vi "试验判定.vi"(7 "Result":refnum<vi>, 10 "判定参数":T1, 11 "XY曲线":cluster{"X":dbl[], "Y":dbl[]}[](array[cluster])) -> (2 "判定项长度":i32, 3 "OK？":bool)   [LabVIEW 2020]
uses:
  Global_Variable/A131258.vi
  <userlib>/_MGI/1D Array/MGI Average/MGI Average (DBL[]).vi
panel:
  out "逆向平均值":dbl
  out "正向平均值":dbl
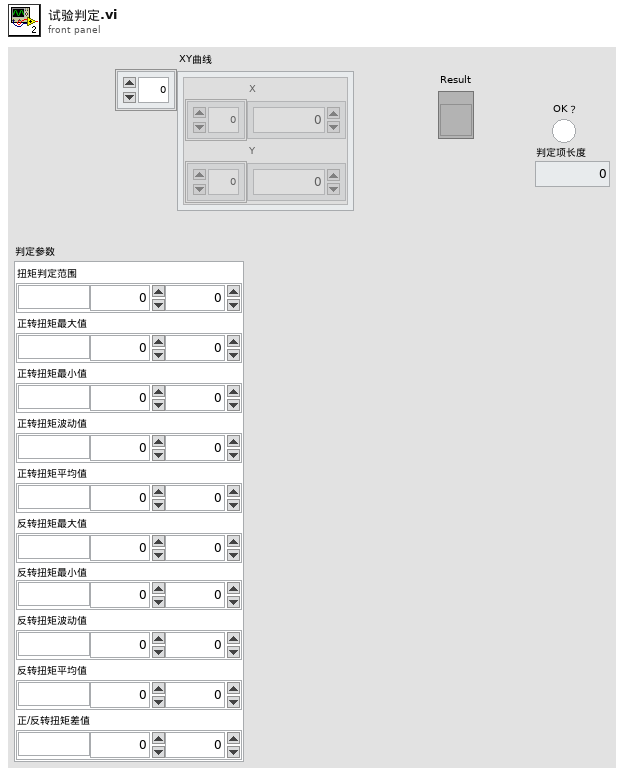
[diagram p1: front panel]
types:
  T1 = cluster{"扭矩判定范围":cluster{"单位":string, "下限":dbl, "上限":dbl}, "正转扭矩最大值":cluster{"单位":string, "下限":dbl, "上限":dbl}, "正转扭矩最小值":cluster{"单位":string, "下限":dbl, "上限":dbl}, "正转扭矩波动值":cluster{"单位":string, "下限":dbl, "上限":dbl}, "正转扭矩平均值":cluster{"单位":string, "下限":dbl, "上限":dbl}, "反转扭矩最大值":cluster{"单位":string, "下限":dbl, "上限":dbl}, "反转扭矩最小值":cluster{"单位":string, "下限":dbl, "上限":dbl}, "反转扭矩波动值":cluster{"单位":string, "下限":dbl, "上限":dbl}, "反转扭矩平均值":cluster{"单位":string, "下限":dbl, "上限":dbl}, "正/反转扭矩差值":cluster{"单位":string, "下限":dbl, "上限":dbl}}
  T2 = cluster{"左平均扭矩":cluster{"正转":dbl, "反转":dbl}, "左矩波动":cluster{"正转":dbl, "反转":dbl}, "左空载":cluster{"正转":dbl, "反转":dbl}, "右平均扭矩":cluster{"正转":dbl, "反转":dbl}, "右扭矩波动":cluster{"正转":dbl, "反转":dbl}, "右空载":cluster{"正转":dbl, "反转":dbl}, "扭矩对称":cluster{"左":dbl, "右":dbl}, "左零点漂移":cluster{"正":dbl, "反":dbl}, "右零点漂移":cluster{"正":dbl, "反":dbl}}
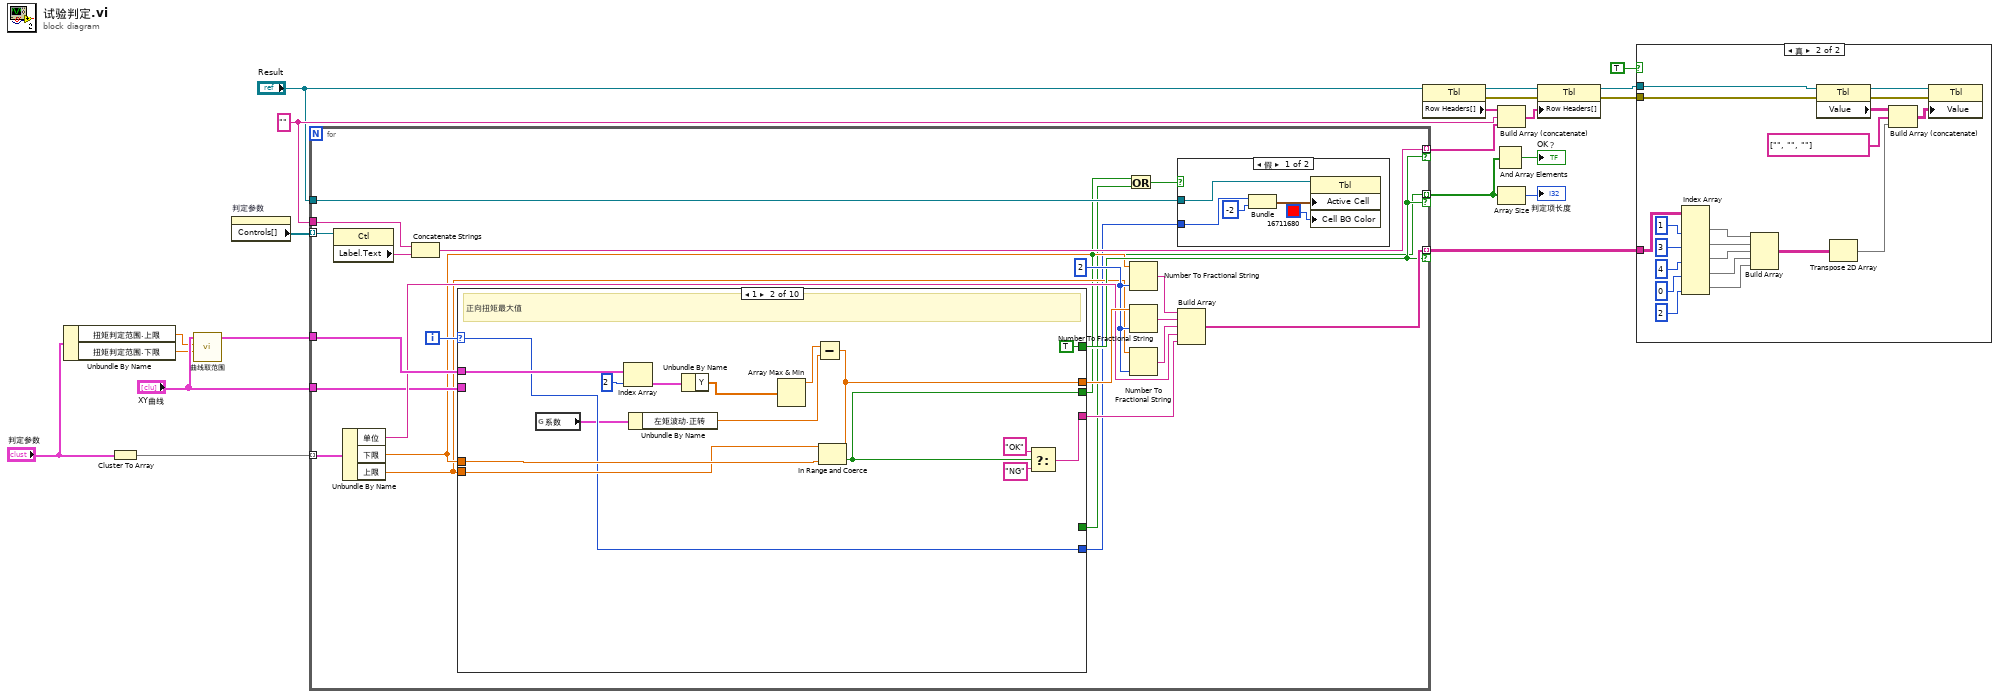
[diagram p0: block diagram]
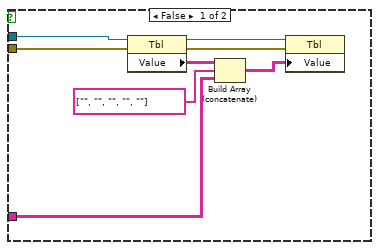
[diagram p2: hidden frame]
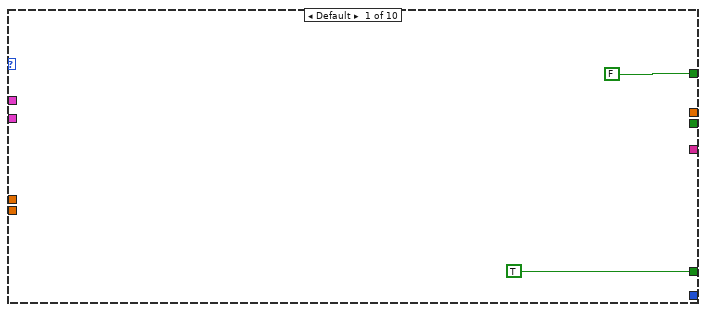
[diagram p4: hidden frame]
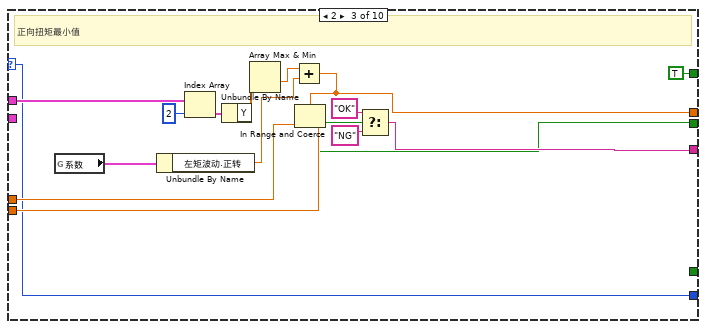
[diagram p5: hidden frame]
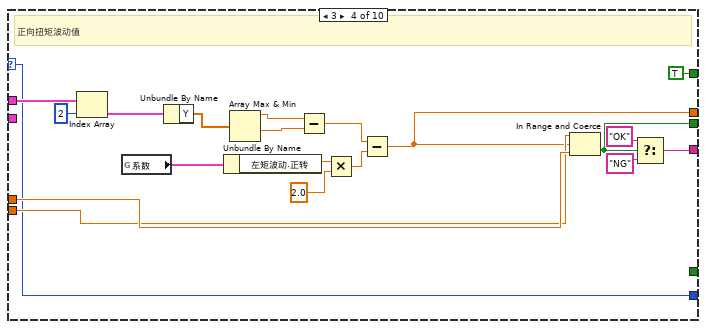
[diagram p6: hidden frame]
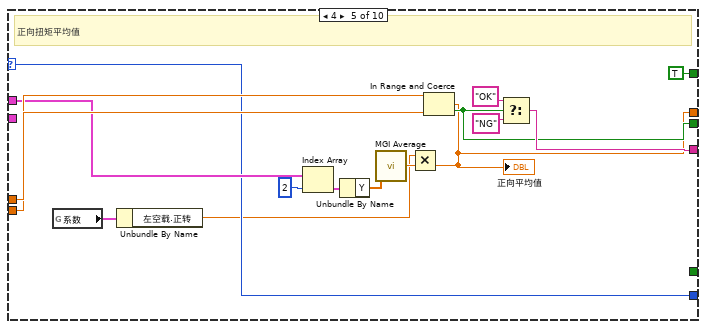
[diagram p7: hidden frame]
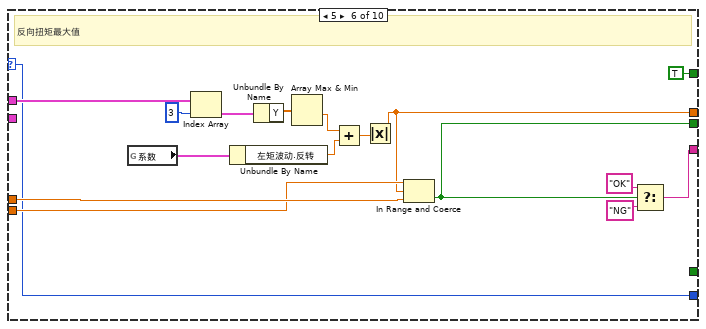
[diagram p8: hidden frame]
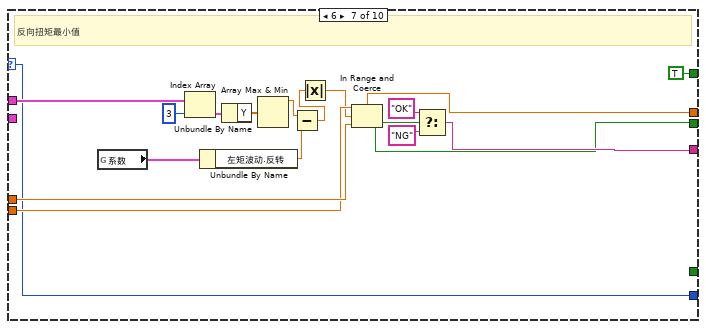
[diagram p9: hidden frame]
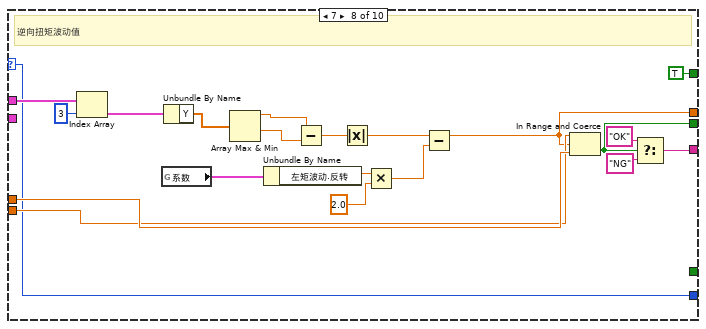
[diagram p10: hidden frame]
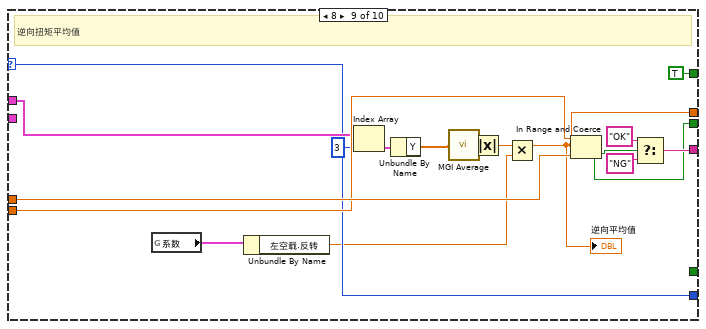
[diagram p11: hidden frame]
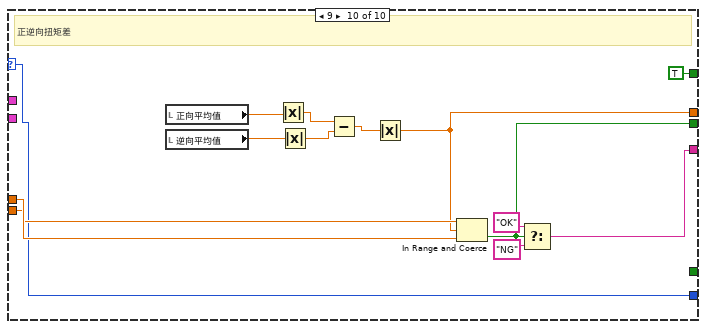
[diagram p12: hidden frame]
diagram:
  w7 = "" ("Label.Text")
  n1 = Unbundle By Name("判定参数") -> ("扭矩判定范围.上限"=w2:dbl, "扭矩判定范围.下限"=w3:dbl)
  n2 = Cluster To Array(cluster="判定参数") -> (array=w21:cluster{"单位":string, "下限":dbl, "上限":dbl}[])
  n3 = call "曲线取范围.vi"("下限"=w3, "上限"=w2, "曲线In"="XY曲线") -> ("曲线Out"=w5:cluster{"X":dbl[], "Y":dbl[]}[])  [unwired: 8 in]
  n4 = property on="判定参数" class="Clust (严格)"() -> ("Controls[]"=w11:refnum<vi>[])  [unwired: 2 in, 2 out]
  n5 = for {
    tunnel: w21 -> [w45] mode=indexing
    tunnel: w11 -> [w43] mode=indexing
    tunnel: w5 -> [w41]
    tunnel: [w25] -> w9 mode=indexing if=w32
    tunnel: [w34] -> w12 mode=indexing if=w32
    tunnel: [w28] -> w14 mode=indexing if=w32
    tunnel: "XY曲线" -> [w31]
    tunnel: w7 -> [w27]
    tunnel: "Result" -> [w26]
    i -> [w44]
    w40 = i16 2 ("精度(6)")
    n6 = property class="Ctl"(reference=w43) -> ("Label.Text"=w33:string)  [unwired: 1 in, 2 out]
    n7 = Unbundle By Name(w45) -> ("单位"=w35:string, "下限"=w30:dbl, "上限"=w29:dbl)
    n8 = Concatenate Strings(w27, w33) -> (w28:string)
    n9 = case shown="1" w44 {
      selector: w44 -> [_ w58 w74 w92 w109 w127 w144 w162 w181 w194]
      tunnel: [_ w53 w69 w85 w106 w121 w138 w159 w177 w195] -> w42
      tunnel: w41 -> [_ w68 w84 w98 w114 w137 w154 w169 w186 _]
      tunnel: [_ w63 w80 w102 w118 w132 w150 w173 w190 w196] -> w36
      tunnel: [_ w57 w73 w91 w108 w126 w143 w160 w179 w193] -> w25
      tunnel: w30 -> [_ w62 w79 w101 w117 w131 w149 w172 w189 w203]
      tunnel: w29 -> [_ w61 w78 w100 w116 w130 w148 w171 w188 w202]
      tunnel: [FALSE TRUE TRUE TRUE TRUE TRUE TRUE TRUE TRUE TRUE] -> w32
      tunnel: w31 -> [_ _ _ _ _ _ _ _ _ _]
      tunnel: [_ w58 w74 w92 w109 w127 w144 w162 w181 w194] -> w24
      tunnel: [TRUE _ _ _ _ _ _ _ _ _] -> w22
      frame Default {
      }
      frame 1 {
        # "正向扭矩最大值"
        n10 = global read "A131258.vi" "系数"() -> (w55:T2)
        n11 = Index Array(array=w68, index=2 ("索引")) -> (element=w66:cluster{"X":dbl[], "Y":dbl[]})
        n12 = Unbundle By Name(w55) -> ("左矩波动.正转"=w54:dbl)
        n13 = Unbundle By Name(w66) -> ("Y"=w59:dbl[])
        n14 = Array Max & Min(array=w59) -> (max value=w56:dbl)  [unwired: 3 out]
        n15 = Subtract(x=w56, y=w54) -> (x-y=w53:dbl)
        n16 = In Range and Coerce(upper limit=w61, x=w53, lower limit=w62) -> (In Range?=w57:bool)  [unwired: 1 out]
        n17 = Select(t="OK", s=w57, f="NG") -> (s? t:f=w63:string)
      }
      frame 2 {
        # "正向扭矩最小值"
        n18 = global read "A131258.vi" "系数"() -> (w71:T2)
        n19 = Unbundle By Name(w71) -> ("左矩波动.正转"=w70:dbl)
        n20 = Index Array(array=w84, index=2 ("索引")) -> (element=w83:cluster{"X":dbl[], "Y":dbl[]})
        n21 = Unbundle By Name(w83) -> ("Y"=w76:dbl[])
        n22 = Array Max & Min(array=w76) -> (min value=w72:dbl)  [unwired: 3 out]
        n23 = Add(x=w72, y=w70) -> (x+y=w69:dbl)
        n24 = In Range and Coerce(upper limit=w78, x=w69, lower limit=w79) -> (In Range?=w73:bool)  [unwired: 1 out]
        n25 = Select(t="OK", s=w73, f="NG") -> (s? t:f=w80:string)
      }
      frame 3 {
        # "正向扭矩波动值"
        n26 = Index Array(array=w98, index=2 ("索引")) -> (element=w97:cluster{"X":dbl[], "Y":dbl[]})
        n27 = global read "A131258.vi" "系数"() -> (w90:T2)
        n28 = Unbundle By Name(w97) -> ("Y"=w95:dbl[])
        n29 = Unbundle By Name(w90) -> ("左矩波动.正转"=w88:dbl)
        n30 = Array Max & Min(array=w95) -> (max value=w94:dbl, min value=w93:dbl)  [unwired: 2 out]
        n31 = Subtract(x=w94, y=w93) -> (x-y=w89:dbl)
        n32 = Multiply(x=w88, y=2.0) -> (x*y=w86:dbl)
        n33 = Subtract(x=w89, y=w86) -> (x-y=w85:dbl)
        n34 = In Range and Coerce(upper limit=w100, x=w85, lower limit=w101) -> (In Range?=w91:bool)  [unwired: 1 out]
        n35 = Select(t="OK", s=w91, f="NG") -> (s? t:f=w102:string)
      }
      frame 4 {
        # "正向扭矩平均值"
        n36 = global read "A131258.vi" "系数"() -> (w107:T2)
        n37 = Unbundle By Name(w107) -> ("左空载.正转"=w105:dbl)
        n38 = Index Array(array=w114, index=2 ("索引")) -> (element=w113:cluster{"X":dbl[], "Y":dbl[]})
        n39 = Unbundle By Name(w113) -> ("Y"=w110:dbl[])
        n40 = call-poly <userlib>:"MGI Average.vi"("Double[]"=w110) -> ("Average"=w111:dbl)  [unwired: 1 in]
        n41 = Multiply(x=w105, y=w111) -> (x*y=w106:dbl)
        "正向平均值" <- w106
        n42 = In Range and Coerce(upper limit=w116, x=w106, lower limit=w117) -> (In Range?=w108:bool)  [unwired: 1 out]
        n43 = Select(t="OK", s=w108, f="NG") -> (s? t:f=w118:string)
      }
      frame 5 {
        # "反向扭矩最大值"
        n44 = global read "A131258.vi" "系数"() -> (w125:T2)
        n45 = Index Array(array=w137, index=3 ("索引")) -> (element=w135:cluster{"X":dbl[], "Y":dbl[]})
        n46 = Unbundle By Name(w125) -> ("左矩波动.反转"=w124:dbl)
        n47 = Unbundle By Name(w135) -> ("Y"=w128:dbl[])
        n48 = Array Max & Min(array=w128) -> (min value=w123:dbl)  [unwired: 3 out]
        n49 = Add(x=w123, y=w124) -> (x+y=w122:dbl)
        n50 = Absolute Value(x=w122) -> (abs(x)=w121:dbl)
        n51 = In Range and Coerce(upper limit=w130, x=w121, lower limit=w131) -> (In Range?=w126:bool)  [unwired: 1 out]
        n52 = Select(t="OK", s=w126, f="NG") -> (s? t:f=w132:string)
      }
      frame 6 {
        # "反向扭矩最小值"
        n53 = global read "A131258.vi" "系数"() -> (w142:T2)
        n54 = Index Array(array=w154, index=3 ("索引")) -> (element=w153:cluster{"X":dbl[], "Y":dbl[]})
        n55 = Unbundle By Name(w142) -> ("左矩波动.反转"=w141:dbl)
        n56 = Unbundle By Name(w153) -> ("Y"=w146:dbl[])
        n57 = Array Max & Min(array=w146) -> (max value=w140:dbl)  [unwired: 3 out]
        n58 = Subtract(x=w140, y=w141) -> (x-y=w139:dbl)
        n59 = Absolute Value(x=w139) -> (abs(x)=w138:dbl)
        n60 = In Range and Coerce(upper limit=w148, x=w138, lower limit=w149) -> (In Range?=w143:bool)  [unwired: 1 out]
        n61 = Select(t="OK", s=w143, f="NG") -> (s? t:f=w150:string)
      }
      frame 7 {
        # "逆向扭矩波动值"
        n62 = Index Array(array=w169, index=3 ("索引")) -> (element=w168:cluster{"X":dbl[], "Y":dbl[]})
        n63 = global read "A131258.vi" "系数"() -> (w158:T2)
        n64 = Unbundle By Name(w168) -> ("Y"=w166:dbl[])
        n65 = Array Max & Min(array=w166) -> (max value=w165:dbl, min value=w164:dbl)  [unwired: 2 out]
        n66 = Unbundle By Name(w158) -> ("左矩波动.反转"=w157:dbl)
        n67 = Subtract(x=w165, y=w164) -> (x-y=w163:dbl)
        n68 = Absolute Value(x=w163) -> (abs(x)=w161:dbl)
        n69 = Multiply(x=w157, y=2.0) -> (x*y=w155:dbl)
        n70 = Subtract(x=w161, y=w155) -> (x-y=w159:dbl)
        n71 = In Range and Coerce(upper limit=w171, x=w159, lower limit=w172) -> (In Range?=w160:bool)  [unwired: 1 out]
        n72 = Select(t="OK", s=w160, f="NG") -> (s? t:f=w173:string)
      }
      frame 8 {
        # "逆向扭矩平均值"
        n73 = global read "A131258.vi" "系数"() -> (w178:T2)
        n74 = Unbundle By Name(w178) -> ("左空载.反转"=w176:dbl)
        n75 = Index Array(array=w186, index=3 ("索引")) -> (element=w185:cluster{"X":dbl[], "Y":dbl[]})
        n76 = Unbundle By Name(w185) -> ("Y"=w184:dbl[])
        n77 = call-poly <userlib>:"MGI Average.vi"("Double[]"=w184) -> ("Average"=w182:dbl)  [unwired: 1 in]
        n78 = Absolute Value(x=w182) -> (abs(x)=w180:dbl)
        n79 = Multiply(x=w180, y=w176) -> (x*y=w177:dbl)
        "逆向平均值" <- w177
        n80 = In Range and Coerce(upper limit=w188, x=w177, lower limit=w189) -> (In Range?=w179:bool)  [unwired: 1 out]
        n81 = Select(t="OK", s=w179, f="NG") -> (s? t:f=w190:string)
      }
      frame 9 {
        # "正逆向扭矩差"
        n82 = local read "正向平均值"() -> (w201:dbl)
        n83 = local read "逆向平均值"() -> (w200:dbl)
        n84 = Absolute Value(x=w201) -> (abs(x)=w199:dbl)
        n85 = Absolute Value(x=w200) -> (abs(x)=w198:dbl)
        n86 = Subtract(x=w199, y=w198) -> (x-y=w197:dbl)
        n87 = Absolute Value(x=w197) -> (abs(x)=w195:dbl)
        n88 = In Range and Coerce(upper limit=w202, x=w195, lower limit=w203) -> (In Range?=w193:bool)  [unwired: 1 out]
        n89 = Select(t="OK", s=w193, f="NG") -> (s? t:f=w196:string)
      }
    }
    n90 = Or(x=w25, y=w22) -> (x .or. y?=w23:bool)
    n91 = Number To Fractional String(number=w30, precision (6)=w40) -> (F-format string=w39:string)  [unwired: 2 in]
    n92 = Number To Fractional String(number=w42, precision (6)=w40) -> (F-format string=w38:string)  [unwired: 2 in]
    n93 = Number To Fractional String(number=w29, precision (6)=w40) -> (F-format string=w37:string)  [unwired: 2 in]
    n94 = case shown="假" w23 {
      tunnel: w26 -> [w50 _]
      tunnel: w24 -> [w46 _]
      frame False {
        n95 = Bundle(w46, -2) -> (w48:cluster{i32, i32})  [unwired: 1 in]
        n96 = property class="Tbl"(reference=w50, "Active Cell"=w48, "Cell BG Color"=u32 16711680 ("活动单元格:单元格背景色")) -> ()  [unwired: 1 in, 2 out]
      }
      frame True {
      }
    }
    n97 = Build Array(w39, w38, w37, w35, w36) -> (w34:string[])
  }
  n98 = property class="Tbl"(reference="Result") -> (reference out=w16:refnum<vi>, error out=w19:errorcluster, "Row Headers[]"=w13:string[])  [unwired: 1 in]
  n99 = And Array Elements(Boolean array=w9) -> (logical AND=→"OK？":bool)
  n100 = Build Array (concatenate)(w13, w7, w14) -> (w15:string[])
  n101 = Array Size(array=w9) -> (size(s)=→"判定项长度":i32)
  n102 = property class="Tbl"(reference=w16, error in=w19, "Row Headers[]"=w15) -> (reference out=w17:refnum<vi>, error out=w18:errorcluster)
  n103 = case shown="真" TRUE {
    tunnel: w18 -> [w212 w232]
    tunnel: w17 -> [w209 w229]
    tunnel: w12 -> [w208 w227]
    frame False {
      n104 = property class="Tbl"(reference=w209, error in=w212) -> (reference out=w210:refnum<vi>, error out=w211:errorcluster, "Value"=w213:string[][])
      n105 = Build Array (concatenate)(w213, string[] ["", "", "", "", ""], w208) -> (w214:string[][])
      n106 = property class="Tbl"(reference=w210, error in=w211, "Value"=w214) -> ()  [unwired: 2 out]
    }
    frame True {
      n107 = Index Array(array=w227, index (col) #1=1 ("禁用的索引 (列)"), index (col) #2=3 ("索引 (列)"), index (col) #3=4 ("索引 (列)"), index (col) #4=0 ("索引 (列)"), index (col) #5=2 ("索引 (列)")) -> (element #1=w223:string[], element #2=w222:string[], element #3=w221:string[], element #4=w216:string[], element #5=w215:string[])  [unwired: 5 in]
      n108 = Build Array(w223, w222, w221, w216, w215) -> (w220:string[][])
      n109 = property class="Tbl"(reference=w229, error in=w232) -> (reference out=w230:refnum<vi>, error out=w231:errorcluster, "Value"=w233:string[][])
      n110 = Transpose 2D Array(2D array=w220) -> (transposed array=w219:string[][])
      n111 = Build Array (concatenate)(w233, string[] ["", "", ""], w219) -> (w234:string[][])
      n112 = property class="Tbl"(reference=w230, error in=w231, "Value"=w234) -> ()  [unwired: 2 out]
    }
  }
